vi "Drive_Teleop.vi"(4 "Joystick_Out":T1) -> ()   [LabVIEW 2019]
uses:
  Utility VIs/Joystick_Controls.ctl
  Subsystems/Drive/Drive_Cluster.ctl
  Subsystems/Drive/Drive_Control_States.ctl
  Subsystems/Drive/Drive_Orientation_States.ctl
  <vilib>/Rock Robotics/WPI/DriverStation/WPI_DriverStationRobotMode2.ctl
  Globals/Drive_Globals.vi
  Robot Global Data.vi
panel:
  in  "sizeOfAverageArray":i32=3
  in  "Rotation Maximum":dbl(slide)=1.0 min=0.3 max=1.0 scale=0.3..1.0
  in  "Rotation Scaling":dbl(slide)=2.0 min=1.0 max=4.0 scale=1.0..4.0
  in  "Rotation Deadband":dbl(slide)=0.05 min=0.0 max=0.25 scale=0.0..0.25
  in  "Strafe Maximum":dbl(slide)=0.5 min=0.3 max=1.0 scale=0.3..1.0
  in  "Strafe Scaling":dbl(slide)=2.0 min=1.0 max=4.0 scale=1.0..4.0
  in  "Strafe Deadband":dbl(slide)=0.05 min=0.0 max=0.25 scale=0.0..0.25
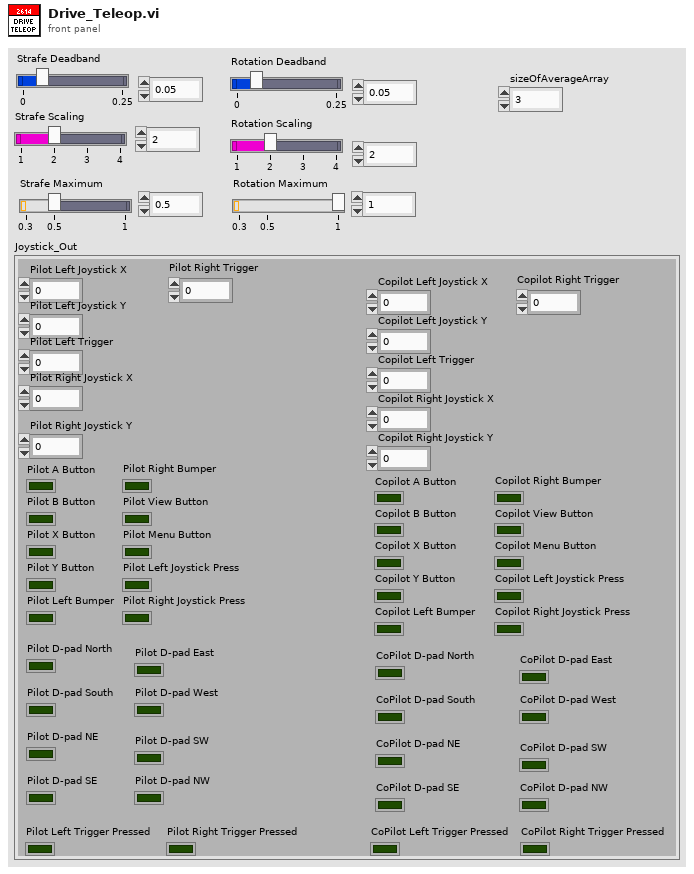
[diagram p1: front panel]
types:
  T1 = typedef "Joystick_Controls.ctl" = cluster{"Pilot Left Joystick X":dbl, "Pilot Left Joystick Y":dbl, "Pilot A Button":bool, "Pilot B Button":bool, "Pilot X Button":bool, "Pilot Y Button":bool, "Pilot Left Bumper":bool, "Pilot Right Bumper":bool, "Pilot View Button":bool, "Pilot Menu Button":bool, "Pilot Left Joystick Press":bool, "Pilot Right Joystick Press":bool, "Pilot Left Trigger":dbl, "Pilot Right Joystick X":dbl, "Pilot Right Joystick Y":dbl, "Pilot Right Trigger":dbl, "Copilot Left Joystick X":dbl, "Copilot Left Joystick Y":dbl, "Copilot A Button":bool, "Copilot B Button":bool, "Copilot X Button":bool, "Copilot Y Button":bool, "Copilot Left Bumper":bool, "Copilot Right Bumper":bool, "Copilot View Button":bool, "Copilot Menu Button":bool, "Copilot Left Joystick Press":bool, "Copilot Right Joystick Press":bool, "Copilot Left Trigger":dbl, "Copilot Right Joystick X":dbl, "Copilot Right Joystick Y":dbl, "Copilot Right Trigger":dbl, "Pilot D-pad North":bool, "Pilot D-pad South":bool, "Pilot D-pad East":bool, "Pilot D-pad West":bool, "Pilot D-pad NE ":bool, "Pilot D-pad SE":bool, "Pilot D-pad SW":bool, "Pilot D-pad NW":bool, "CoPilot D-pad North":bool, "CoPilot D-pad South":bool, "CoPilot D-pad East":bool, "CoPilot D-pad West":bool, "CoPilot D-pad NE":bool, "CoPilot D-pad SE":bool, "CoPilot D-pad SW":bool, "CoPilot D-pad NW":bool, "Pilot Left Trigger Pressed":bool, "Pilot Right Trigger Pressed":bool, "CoPilot Left Trigger Pressed":bool, "CoPilot Right Trigger Pressed":bool}
  T2 = typedef "WPI_DriverStationRobotMode2.ctl" = enum16{"Autonomous Disabled", "Autonomous Enabled", "Teleop Disabled", "Teleop Enabled", "Disconnected", "Finish", "Test Disabled", "Test Enabled", "Emergency Stopped"}
  T3 = typedef "Drive_Cluster.ctl" = cluster{"Control_State":T4, "Vertical_Throttle":dbl, "Lateral_Throttle":dbl, "Rotational_Throttle":dbl, "Strafe_In_Deadband":bool, "Rotation_In_Deadband":bool, "Orientation_State":T5, "Parameters":dbl[], "Step":i32, "Auto_Notifier":refnum<notifier>}
  T4 = typedef "Drive_Control_States.ctl" = enum16{"No-Op", "Manual_Control", "Command_DriveDistanceAtAngle", ""}
  T5 = typedef "Drive_Orientation_States.ctl" = enum16{"Robot-Oriented", "Field-Oriented"}
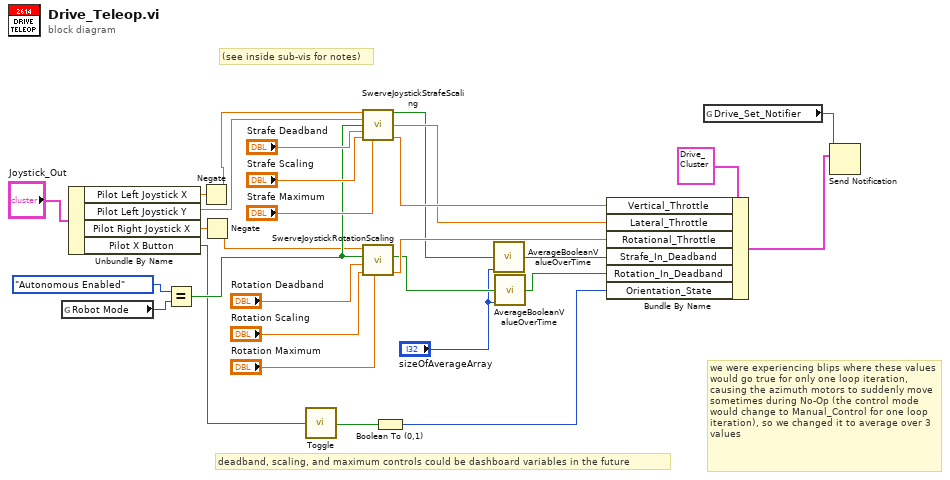
[diagram p0: block diagram]
diagram:
  # "we were experiencing blips where these values would go true for only one loop iteration, causing the azimuth motors to suddenly move sometimes during No-Op (the control mode would change to Manual_Control for one loop iteration), so we changed it to average over 3 values"
  # "(see inside sub-vis for notes)"
  # "deadband, scaling, and maximum controls could be dashboard variables in the future"
  n1 = global read "Robot Global Data.vi" "Robot Mode"() -> (w17:T2)
  n2 = Unbundle By Name("Joystick_Out") -> ("Pilot Left Joystick X"=w10:dbl, "Pilot Left Joystick Y"=w9:dbl, "Pilot Right Joystick X"=w25:dbl, "Pilot X Button"=w12:bool)
  n3 = Equal?(x=WPI_DriverStationRobotMode2."Autonomous Enabled" ("Robot Mode"), y=w17) -> (x = y?=w16:bool)
  n4 = Negate(x=w10) -> (-x=w8:dbl)
  n5 = Negate(x=w25) -> (-x=w7:dbl)
  n6 = call "Toggle.vi"("Boolean"=w12) -> ("Boolean Out"=w11:bool)
  n7 = call "SwerveJoystickStrafeScaling.vi"("Raw Joystick X"=w8, "Raw Joystick Y"=w9, "Auto Control"=w16, "Strafe Deadband"="Strafe Deadband", "Strafe Scaling"="Strafe Scaling", "Strafe Maximum"="Strafe Maximum") -> ("In Deadband"=w6:bool, "Scaled Joystick X"=w14:dbl, "Scaled Joystick Y"=w15:dbl)  [unwired: 7 in]
  n8 = call "SwerveJoystickRotationScaling.vi"("Rotation Maximum"="Rotation Maximum", "Rotation Scaling"="Rotation Scaling", "Rotation Deadband"="Rotation Deadband", "Auto Control"=w16, "Raw Joystick Rotation"=w7) -> ("Scaled Joystick Rotation"=w13:dbl, "In Deadband"=w4:bool)  [unwired: 4 in]
  n9 = Boolean To (0,1)(Boolean=w11) -> (0, 1=w1:i16)
  n10 = call "AverageBooleanValueOverTime.vi"("input boolean"=w6, "sizeOfAverageArray (5)"="sizeOfAverageArray") -> ("averaged"=w5:bool)  [unwired: 13 in]
  n11 = call "AverageBooleanValueOverTime.vi"("input boolean"=w4, "sizeOfAverageArray (5)"="sizeOfAverageArray") -> ("averaged"=w3:bool)  [unwired: 13 in]
  n12 = Bundle By Name(cluster=T3 {"Control_State"=enum."Manual_Control", "Vertical_Throttle"=0.0, "Lateral_Throttle"=0.0, "Rotational_Throttle"=0.0, "Strafe_In_Deadband"=FALSE, "Rotation_In_Deadband"=FALSE, "Orientation_State"=enum."Robot-Oriented", "Parameters"=[], "Step"=0, "Auto_Notifier"=refnum} ("notification"), "Vertical_Throttle"=w15, "Lateral_Throttle"=w14, "Rotational_Throttle"=w13, "Strafe_In_Deadband"=w5, "Rotation_In_Deadband"=w3, "Orientation_State"=w1) -> (w29:T3)
  n13 = global read "Drive_Globals.vi" "Drive_Set_Notifier"() -> (w26:refnum<notifier>)
  n14 = Send Notification(notification=w29, notifier=w26) -> ()  [unwired: 1 in, 2 out]
